vi "niFpgaHtCmulSimDfxpTemplate.vi"(0 "xr":fxp<+/-,31,31>, 5 "xi":fxp<+/-,31,31>, 7 "yr":fxp<+/-,31,31>, 9 "yi":fxp<+/-,31,31>, 11 "input valid":bool=TRUE, 12 "ready for output":bool=TRUE) -> (4 "pr":fxp<+/-,63,63>, 6 "pi":fxp<+/-,63,63>, 10 "overflow":bool, 14 "ready for input":bool, 15 "output valid":bool)   [LabVIEW 2017]
uses:
  <vilib>/rvi/FXPMathLib/SharedSubVIs/typedef/nifxpmath_BASIC_ImplementationSettings.ctl
  <vilib>/fxp/LVFixedPointQuantizationPolicyTypeDef.ctl
  <vilib>/fxp/LVFixedPointOverflowPolicyTypeDef.ctl
  <vilib>/rvi/ClientSDK/Core/DevComputerLib/Private/Dfxp64.ctl
  <vilib>/fxp/LVFixedPointRepBitsTypeDef.ctl
  <vilib>/rvi/ClientSDK/Core/DevComputerLib/Private/Dfxp64OutputConfig.ctl
  <vilib>/rvi/ClientSDK/Core/DevComputerLib/niFpgaDevCompUtilities.lvlib
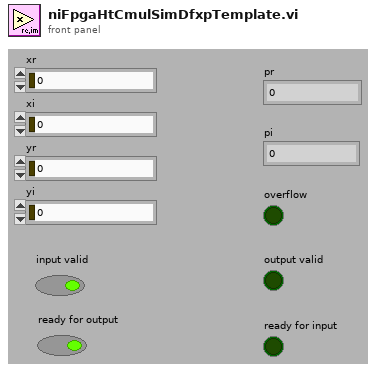
[diagram p1: front panel]
types:
  T1 = typedef "niFpgaDevCompUtilities.lvlib/Dfxp64OutputConfig.ctl" = cluster{"representation":T2, "rounding mode":T3, "overflow mode":T4}
  T2 = typedef "LVFixedPointRepBitsTypeDef.ctl" = cluster{"Signed":bool, "Word Length":u32, "Integer Word Length":i32}
  T3 = typedef "LVFixedPointQuantizationPolicyTypeDef.ctl" = enum32{"Truncate", "Round-Half-Up (Asymmetric)", "Round-Half-Even"}
  T4 = typedef "LVFixedPointOverflowPolicyTypeDef.ctl" = enum32{"Wrap", "Saturate"}
  T5 = typedef "niFpgaDevCompUtilities.lvlib/Dfxp64.ctl" = cluster{"int64":fxp<+/-,64,64>, "representation":T2}
  T6 = typedef "nifxpmath_BASIC_ImplementationSettings.ctl" = cluster{"NumOfStages":i32, "SupportSCTL":bool, "InputRegister":bool, "OutputRegister":bool, "rounding mode":T3, "overflow mode":T4}
  T7 = typedef "niFpgaDevCompUtilities.lvlib/Cint64.ctl" = cluster{"real":i64, "imag":i64, "pr ovfl":bool, "pi ovfl":bool, "op ovfl":bool}
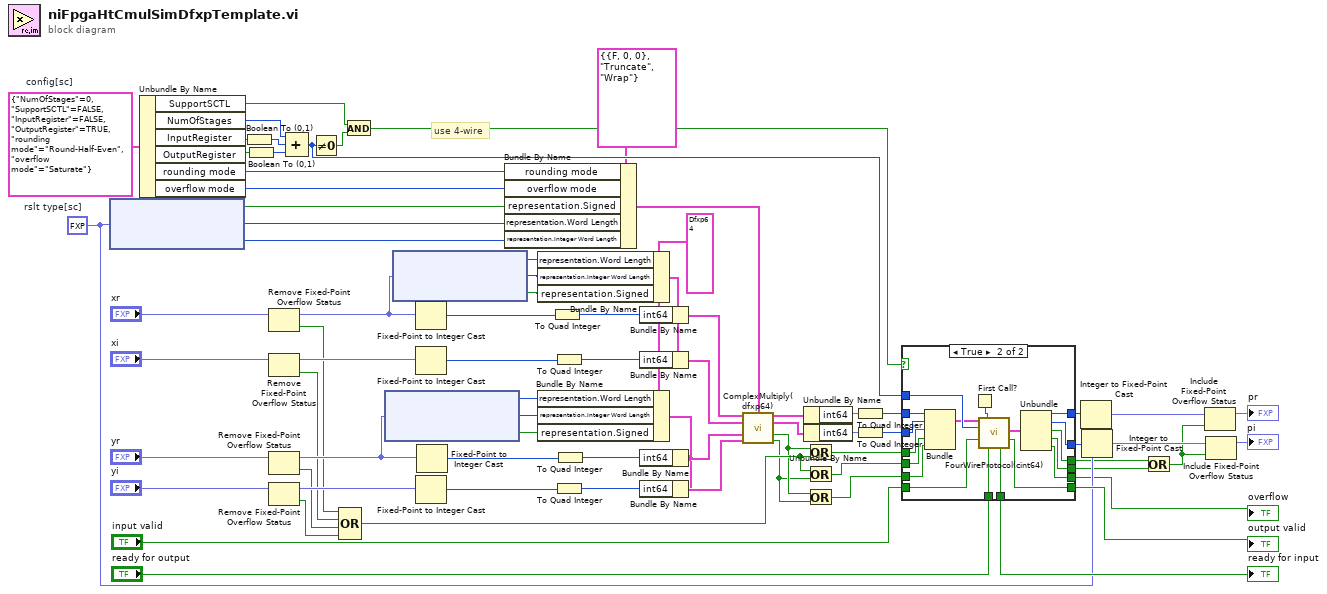
[diagram p0: block diagram]
diagram:
  w16 = T5 {"int64"=0.0, "representation"={"Signed"=FALSE, "Word Length"=0, "Integer Word Length"=0}} ("dfxp")
  w47 = fxp<+/-,63,63> 0.0  # rslt type[sc]
  w72 = T6 {"NumOfStages"=0, "SupportSCTL"=FALSE, "InputRegister"=FALSE, "OutputRegister"=TRUE, "rounding mode"=enum."Round-Half-Even", "overflow mode"=enum."Saturate"}  # config[sc]
  # "use 4-wire"
  n1 = node(w47) -> (w44:bool, w43:u32, w42:i32)
  n2 = Unbundle By Name(w72) -> ("SupportSCTL"=w71:bool, "NumOfStages"=w50:i32, "InputRegister"=w52:bool, "OutputRegister"=w51:bool, "rounding mode"=w46:T3, "overflow mode"=w45:T4)
  n3 = Boolean To (0,1)(Boolean=w52) -> (0, 1=w54:i16)
  n4 = Boolean To (0,1)(Boolean=w51) -> (0, 1=w53:i16)
  n5 = Remove Fixed-Point Overflow Status(3:"xr") -> (0:w62:bool, 1:w63:fxp<+/-,31,31>)
  n6 = Remove Fixed-Point Overflow Status(3:"xi") -> (0:w61:bool, 1:w64:fxp<+/-,31,31>)
  n7 = Remove Fixed-Point Overflow Status(3:"yr") -> (0:w60:bool, 1:w65:fxp<+/-,31,31>)
  n8 = Remove Fixed-Point Overflow Status(3:"yi") -> (0:w59:bool, 1:w66:fxp<+/-,31,31>)
  n9 = Compound Arithmetic op=unknown(w50, w54, w53) -> (w48:i32)
  n10 = Not Equal To 0?(x=w48) -> (x != 0?=w49:bool)
  n11 = Compound Arithmetic op=OR(w62, w61, w60, w59) -> (w41:bool)
  n12 = And(x=w71, y=w49) -> (x .and. y?=w70:bool)
  n13 = node(w65) -> (w1:u32, w19:i32, w18:bool)
  n14 = node(w63) -> (w2:u32, w21:i32, w22:bool)
  n15 = Fixed-Point to Integer Cast(1:w63) -> (0:w10:i32)
  n16 = Fixed-Point to Integer Cast(1:w64) -> (0:w11:i32)
  n17 = Fixed-Point to Integer Cast(1:w66) -> (0:w13:i32)
  n18 = Fixed-Point to Integer Cast(1:w65) -> (0:w12:i32)
  n19 = Bundle By Name(cluster=T1 {"representation"={"Signed"=FALSE, "Word Length"=0, "Integer Word Length"=0}, "rounding mode"=enum."Truncate", "overflow mode"=enum."Wrap"} ("kP"), "rounding mode"=w46, "overflow mode"=w45, "representation.Signed"=w44, "representation.Word Length"=w43, "representation.Integer Word Length"=w42) -> (w8:T1)
  n20 = Bundle By Name(cluster=w16, "representation.Word Length"=w2, "representation.Integer Word Length"=w21, "representation.Signed"=w22) -> (w20:T5)
  n21 = Bundle By Name(cluster=w16, "representation.Word Length"=w1, "representation.Integer Word Length"=w19, "representation.Signed"=w18) -> (w17:T5)
  n22 = To Quad Integer(1:w10) -> (0:w30:i64)
  n23 = To Quad Integer(1:w11) -> (0:w31:i64)
  n24 = To Quad Integer(1:w13) -> (0:w33:i64)
  n25 = To Quad Integer(1:w12) -> (0:w34:i64)
  n26 = Bundle By Name(cluster=w20, "int64"=w30) -> (w28:T5)
  n27 = Bundle By Name(cluster=w20, "int64"=w31) -> (w29:T5)
  n28 = Bundle By Name(cluster=w17, "int64"=w34) -> (w32:T5)
  n29 = Bundle By Name(cluster=w17, "int64"=w33) -> (w27:T5)
  n30 = call <vilib>:"ComplexMultiply(dfxp64).vi"("xr"=w28, "output config"=w8, "xi"=w29, "yr"=w32, "yi"=w27) -> ("pr"=w15:T5, "pi"=w14:T5, "overflow pr"=w7:bool, "overflow pi"=w6:bool)  [unwired: 7 in]
  n31 = Unbundle By Name(w15) -> ("int64"=w36:fxp<+/-,64,64>)
  n32 = Unbundle By Name(w14) -> ("int64"=w35:fxp<+/-,64,64>)
  n33 = Or(x=w7, y=w41) -> (x .or. y?=w5:bool)
  n34 = Or(x=w41, y=w6) -> (x .or. y?=w4:bool)
  n35 = Or(x=w7, y=w6) -> (x .or. y?=w3:bool)
  n36 = To Quad Integer(1:w36) -> (0:w26:i64)
  n37 = To Quad Integer(1:w35) -> (0:w25:i64)
  n38 = case shown="True" w70 {
    tunnel: w26 -> [w81 w100]
    tunnel: w25 -> [w82 w99]
    tunnel: "input valid" -> [_ w98]
    tunnel: [w81 w96] -> w24
    tunnel: [w82 w95] -> w23
    tunnel: "ready for output" -> [_ w94]
    tunnel: [_ w93] -> w74
    tunnel: [_ w92] -> w73
    tunnel: w48 -> [_ w90]
    tunnel: w4 -> [w79 w87]
    tunnel: [w80 w89] -> w39
    tunnel: w5 -> [w80 w88]
    tunnel: w3 -> [w78 w86]
    tunnel: [w79 w84] -> w38
    tunnel: [w78 w83] -> w40
    frame False {
    }
    frame True {
      n39 = Bundle(w100, w99, w88, w87, w86) -> (w85:cluster{i64, i64, bool, bool, bool})  [unwired: 1 in]
      n40 = First Call?() -> (First Call?: T/F=w91:bool)
      n41 = call <vilib>:"FourWireProtocol(cint64).vi"("complex data in"=w85, "reset"=w91, "latency (1)"=w90, "input valid"=w98, "ready for output"=w94) -> ("complex data out"=w97:T7, "output valid"=w92:bool, "ready for input"=w93:bool)  [unwired: 7 in, 1 out]
      n42 = Unbundle(w97) -> ("real"=w96:i64, "imag"=w95:i64, "pr ovfl"=w89:bool, "pi ovfl"=w84:bool, "op ovfl"=w83:bool)
    }
  }
  "output valid" <- w73
  "ready for input" <- w74
  "overflow" <- w40
  n43 = Integer to Fixed-Point Cast(fixed-point type=w47, integer=w24) -> (fixed-point=w58:fxp<+/-,63,63>)
  n44 = Integer to Fixed-Point Cast(fixed-point type=w47, integer=w23) -> (fixed-point=w56:fxp<+/-,63,63>)
  n45 = Or(x=w39, y=w38) -> (x .or. y?=w37:bool)
  n46 = Include Fixed-Point Overflow Status(2:w37, 3:w58) -> (1:→"pr":fxp<+/-,63,63>)
  n47 = Include Fixed-Point Overflow Status(2:w37, 3:w56) -> (1:→"pi":fxp<+/-,63,63>)
